vi "SSM from Feedforward Gains.vi"(8 "dt":dbl=-1.0, 10 "kA":dbl, 11 "kV":dbl) -> (3 "Continious State Space Model":T1)   [LabVIEW 2020]
uses:
  CB State Space.ctl
  <vilib>/Analysis/Matrix/Datatypes/RealMatrix.ctl
  <vilib>/Analysis/Matrix/NI_Matrix.lvlib
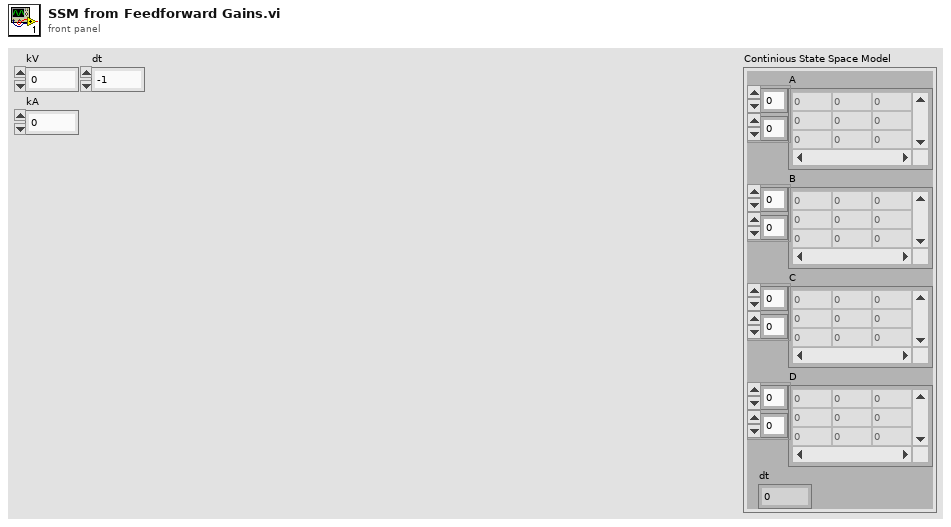
[diagram p1: front panel]
types:
  T1 = typedef "CB State Space.ctl" = cluster{"A":T2, "B":T2, "C":T2, "D":T2, "dt":dbl}
  T2 = typedef "NI_Matrix.lvlib/RealMatrix.ctl" = dbl[][]
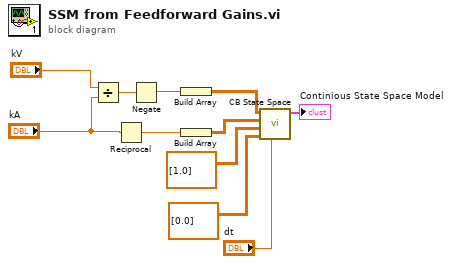
[diagram p0: block diagram]
diagram:
  n1 = Divide(x="kV", y="kA") -> (x/y=w9:dbl)
  n2 = Reciprocal(x="kA") -> (1/x=w7:dbl)
  n3 = Negate(x=w9) -> (-x=w8:dbl)
  n4 = Build Array(w8) -> (w6:T2)
  n5 = Build Array(w7) -> (w5:T2)
  n6 = call "CB State Space.vi"("dt"="dt", "D"=T2 [[0.0]], "C"=T2 [[1.0]], "B"=w5, "A"=w6) -> ("State Space Model"=→"Continious State Space Model":T1)  [unwired: 5 in, 1 out]
